vi "subvi Robot Wait for Character.vi"(2 "error in":errorcluster, 3 "VISA In":refnum<visa-resource-name>) -> (0 "error out":errorcluster, 1 "VISA Out":refnum<visa-resource-name>)   [LabVIEW 2012]
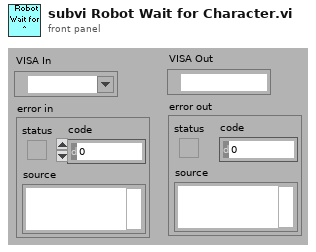
[diagram p1: front panel]
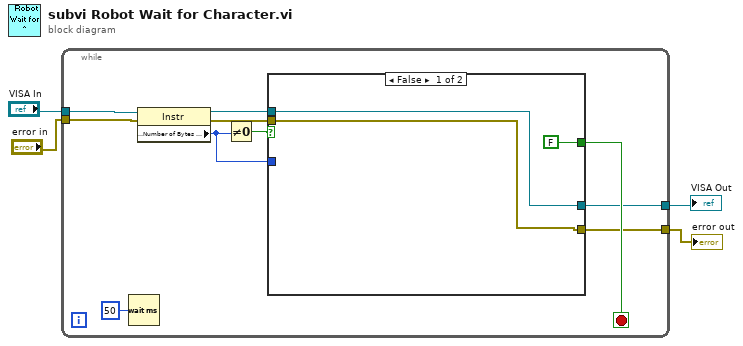
[diagram p0: block diagram]
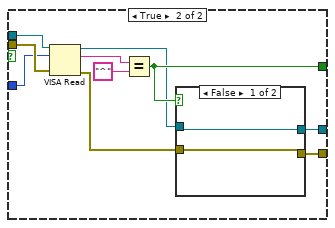
[diagram p2: hidden frame]
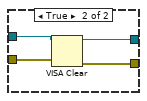
[diagram p3: hidden frame]
diagram:
  n1 = while {
    tunnel: [w8] -> w2
    tunnel: [w7] -> w1
    tunnel: "VISA In" -> [w6]
    tunnel: "error in" -> [w5]
    stop <- w9 stop-if-true
    n2 = Wait (ms)(milliseconds to wait=u32 50) -> ()  [unwired: 1 out]
    n3 = property class="Instr"(reference=w6, error in=w5) -> (reference out=w12:refnum<visa-resource-name>, error out=w11:errorcluster, "Serial Settings:Number of Bytes at Serial Port"=w10:u32)
    n4 = Not Equal To 0?(x=w10) -> (x != 0?=w13:bool)
    n5 = case shown="False" w13 {
      tunnel: w12 -> [w16 w27]
      tunnel: w11 -> [w15 w26]
      tunnel: w10 -> [_ w25]
      tunnel: [FALSE w22] -> w9
      tunnel: [w16 w19] -> w8
      tunnel: [w15 w18] -> w7
      frame False {
      }
      frame True {
        n6 = VISA Read(VISA resource name=w27, byte count=w25, error in (no error)=w26) -> (VISA resource name out=w20:refnum<visa-resource-name>, read buffer=w24:string, error out=w21:errorcluster)  [unwired: 1 out]
        n7 = Equal?(x=w24, y="^") -> (x = y?=w22:bool)
        n8 = case shown="False" w22 {
          tunnel: w20 -> [w28 w33]
          tunnel: w21 -> [w29 w32]
          tunnel: [w28 w31] -> w19
          tunnel: [w29 w30] -> w18
          frame False {
          }
          frame True {
            n9 = VISA Clear(VISA resource name=w33, error in (no error)=w32) -> (VISA resource name out=w31:refnum<visa-resource-name>, error out=w30:errorcluster)
          }
        }
      }
    }
  }
  "VISA Out" <- w2
  "error out" <- w1
